vi "XIPIN_AXI_Interrupt_Controller_4_1.vi"   [LabVIEW 2017]
doc: "The LogiCORE IP AXI Interrupt Controller (AXI INTC) core concentrates multiple interrupt inputs from peripheral devices to a single interrupt output to the system processor.\n------------------------------------\n<b>Need License</b> : No\n<b>Interface</b> : AXI4"
uses:
  <vilib>/rvi/XilinxIP/XIPIN_XNode/niFpgaXIPIN.xnode
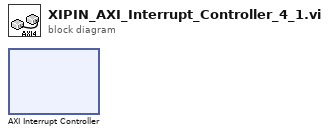
[diagram p0: block diagram]
diagram:
  n1 = xnode ("AXI Interrupt Controller")() -> ()
